vi "CalculateDependencies.vi"(6 "additional included files":path[](array[path]), 8 "error in (no error)":errorcluster, 11 "Build in":refnum<class "AB_EXE.lvclass">) -> (0 "error out":errorcluster, 2 "Dependencies":T1[](array[typedef]), 3 "Build out":refnum<class "AB_EXE.lvclass">)   [LabVIEW 2020, in "AB_EXE.lvclass"]
uses:
  <vilib>/AppBuilder/AB_Classes/EXE/AB_EXE.lvclass
  e:/builds/penguin/labview/branches/2020/dev/dist/vi.lib/AppBuilder/AB_Classes/Build/AB_Build.lvclass
  <vilib>/AppBuilder/AB_Dependency.ctl
  <vilib>/Utility/lvfile.llb/LVFileType.ctl
  <vilib>/AppBuilder/AB_Classes/EXE/AB_EXE.lvclass/AB_EXE.ctl
  <vilib>/AppBuilder/AB_Classes/EXE/AB_EXE_SharedVar_LibInfo.ctl
  <vilib>/AppBuilder/AB_Classes/Application/AB_Application.lvclass
  <vilib>/AppBuilder/AB_Classes/Build/AB_Build.lvclass
  <vilib>/Utility/lvfile.llb/NI_FileType.lvlib
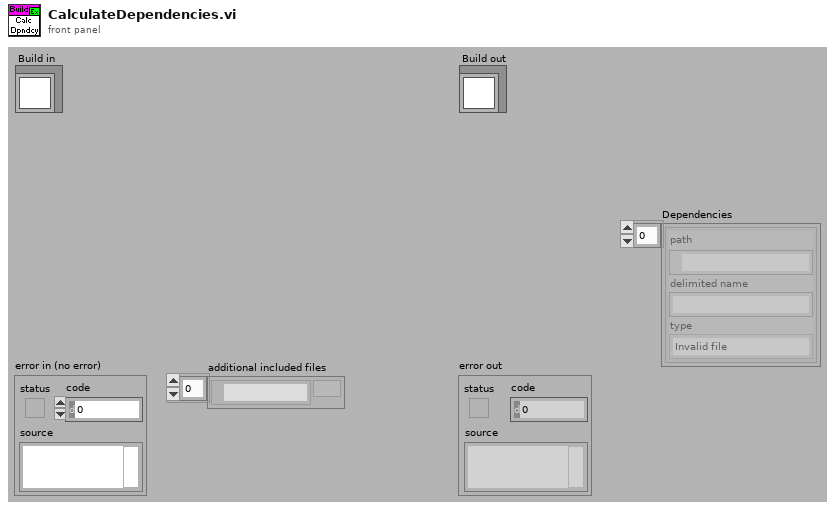
[diagram p1: front panel]
types:
  T1 = typedef "AB_Dependency.ctl" = cluster{"path":path, "delimited name":string, "type":T2}
  T2 = typedef "NI_FileType.lvlib/LVFileType.ctl" = enum32{"Invalid file", "Unknown type", "Instrument", "Control", "Polymorphic VI", "Project", "Library", "LVClass", "XControl", "XNode", "Shared library", ".NET assembly", "ActiveX interface", "CIN", "Run-time menu", "Palette menu", "Help file", "LLB", "XNode Edit Dependency", "Class Private Data Control", "Statechart", "MathScript .m file", "Ladder Diagram", "LVLibp", "XNode Build Dependency"}
  T3 = typedef "AB_EXE_SharedVar_LibInfo.ctl" = cluster{"LibraryPath":path, "LibraryItemID":string, "target":string, "deploy":bool}
  T4 = typedef "AB_Build.ctl" = cluster{"buildSpecName":string, "buildSpecDescription":string, "destinations":refnum<class "AB_Destination.lvclass">[], "exclusionOption":T5, "defaultLanguage":string, "supportedLanguages":string[], "excludedDirectories":path[], "buildContext":refnum<vi>, "buildObject":T6, "preview":bool, "programatic":bool, "progressBarEvents":T7, "userLog_Path":path, "preActionID":string, "preAction_Path":path, "postActionID":string, "postAction_Path":path, "eng_checkForBrokenVIs?":bool, "eng_verboseLinkerErrors?":bool, "localDest_Path":path, "targetDest_Path":path, "removeVIObject":u16, "cache":refnum<class "PreviewCache.lvclass">, "use cache":bool, "previewCache_ID":string, "buildCache_ID":string, "eng_TempLocalDest_Path":path, "eng_collectDependencies?":bool, "versionInfo":cluster{"buildVersion":cluster{"major":u16, "minor":u16, "patch":u16, "build":u16}, "autoIncrement":bool}, "eng_enableVIChecksums":bool}
  T5 = typedef "AB_Exclusion_Option.ctl" = cluster{"typedefs":bool, "polymorphicVIs":bool, "unusedLibraryItems":bool, "modifyLibraryFile":bool, "edit-timeDependencies":bool, "inlineVIs":bool, "dependent PPLs":bool, "dependent DLLs":bool}
  T6 = typedef "ItemRef.ctl" = u64
  T7 = typedef "provcom_ProgressBar_Events.ctl" = cluster{"newJob":refnum<user-event>, "newItem":refnum<user-event>, "errorMsg":T8, "cancel":refnum<user-event>}
  T8 = typedef "mxLvBuildError.ctl" = refnum<user-event>
  T9 = typedef "AB_Engine_RTDEP_Dep_Lib_Info.ctl" = cluster{"Library Path":path, "Target Name":string}
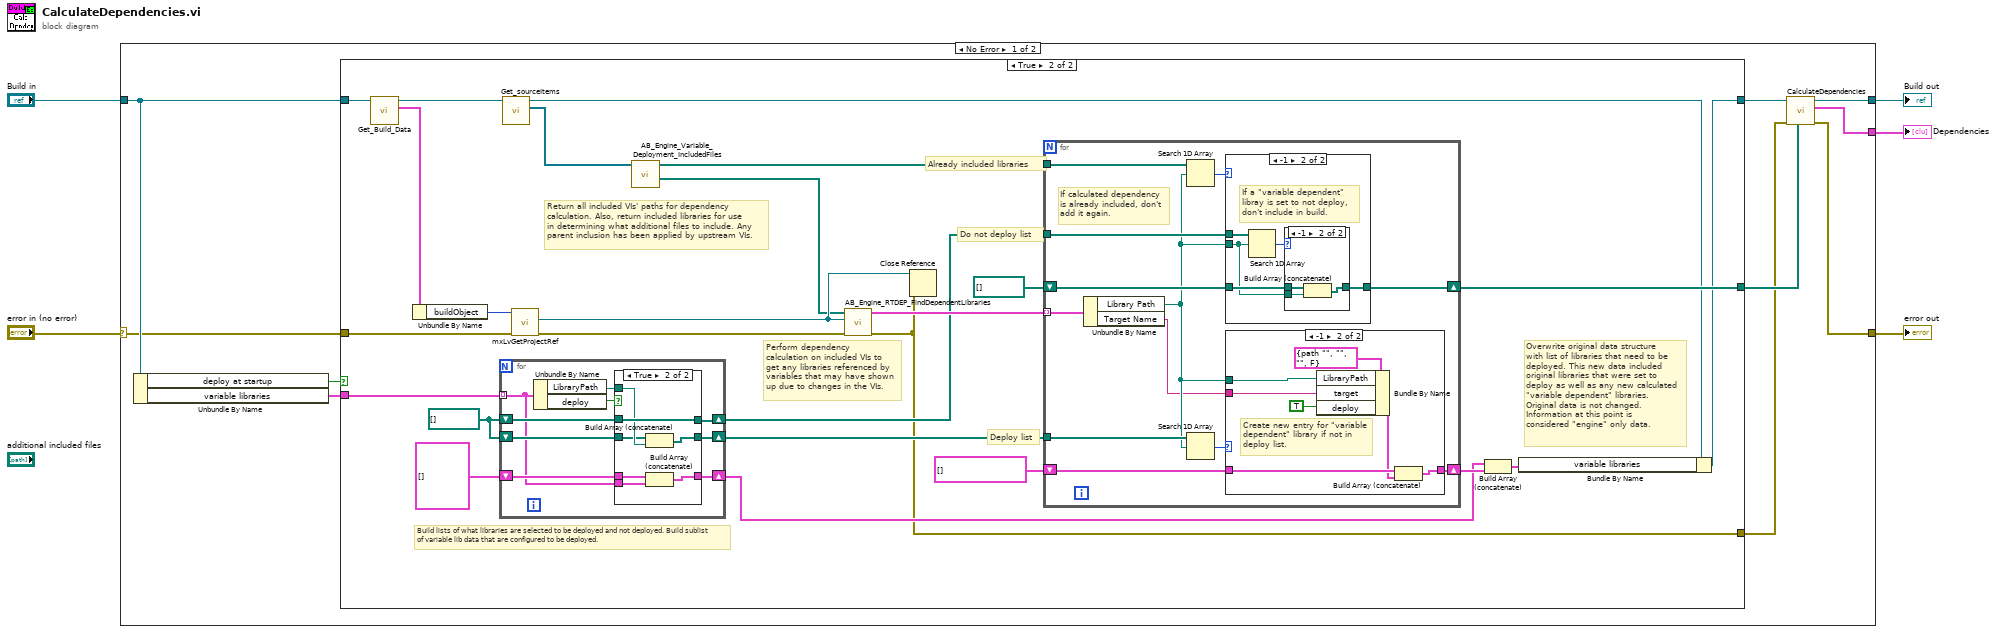
[diagram p0: block diagram]
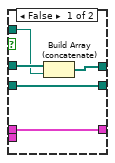
[diagram p3: hidden frame]
diagram:
  n1 = case shown="No Error" "error in (no error)" {
    selector: "error in (no error)" -> [w7 w95]
    tunnel: [w15 w95] -> w5
    tunnel: [w14 w94] -> w4
    tunnel: "Build in" -> [w12 w94]
    tunnel: [w6 _] -> w1
    frame No Error {
      n2 = Unbundle By Name(w12) -> ("deploy at startup"=w13:bool, "variable libraries"=w10:T3[])
      n3 = case shown="True" w13 {
        tunnel: w12 -> [w17 w42]
        tunnel: [w17 w28] -> w11
        tunnel: w10 -> [_ w26]
        tunnel: [_ w36] -> w9
        tunnel: w7 -> [w16 w23]
        tunnel: [w16 w18] -> w8
        frame False {
        }
        frame True {
          w34 = path[] []
          # "Overwrite original data structure with list of libraries that need to be deployed. This new data included original libraries that were set to deploy as well as any new calculated \"variable dependent\" libraries. Original data is not changed. Information at this point is considered \"engine\" only data."
          # "Already included libraries"
          # "Return all included VIs' paths for dependency calculation. Also, return included libraries for use in determining what additional files to include. Any parent inclusion has been applied by upstream VIs."
          # "Perform dependency calculation on included VIs to get any libraries referenced by variables that may have shown up due to changes in the VIs."
          # "Build lists of what libraries are selected to be deployed and not deployed. Build sublist of variable lib data that are configured to be deployed."
          # "Do not deploy list"
          # "Deploy list"
          n4 = call <vilib>:"Get_Build_Data.vi"("Class in"=w42) -> ("data"=w40:T4, "Class out"=w41:refnum<class "AB_EXE.lvclass">)  [unwired: 1 in, 8 out]
          n5 = Unbundle By Name(w40) -> ("buildObject"=w39:T6)
          n6 = for {
            tunnel: w26 -> [w43] mode=indexing
            shift-right: [w50] -> w37
            shift-left: w34 -> [w49]
            shift-right: [w48] -> w33
            shift-left: w34 -> [w47]
            shift-right: [w44] -> w25
            shift-left: T3[] [] ("variable libraries") -> [w45]
            n7 = Unbundle By Name(w43) -> ("LibraryPath"=w46:path, "deploy"=w51:bool)
            n8 = case shown="True" w51 {
              tunnel: [w56 w63] -> w50
              tunnel: w49 -> [w55 w63]
              tunnel: w46 -> [w54 w62]
              tunnel: [w53 w61] -> w48
              tunnel: w47 -> [w53 w60]
              tunnel: w45 -> [w52 w59]
              tunnel: [w52 w58] -> w44
              tunnel: w43 -> [_ w57]
              frame False {
                n9 = Build Array (concatenate)(w55, w54) -> (w56:path[])
              }
              frame True {
                n10 = Build Array (concatenate)(w60, w62) -> (w61:path[])
                n11 = Build Array (concatenate)(w59, w57) -> (w58:T3[])
              }
            }
          }
          n12 = call <vilib>:"Get_sourceItems.vi"("Class in"=w41) -> ("sourceItems"=w21:refnum<class "AB_Source.lvclass">[], "Class out"=w29:refnum<class "AB_EXE.lvclass">)  [unwired: 1 in, 8 out]
          n13 = call <resource>:"mxLvGetProjectRef.vi"("error in"=w23, "Item"=w39) -> ("error out"=w22:errorcluster, "Project Refnum"=w35:refnum<vi>)  [unwired: 8 out]
          n14 = call <vilib>:"AB_Engine_Variable_Deployment_IncludedFiles.vi"("source items"=w21) -> ("Included VIs"=w19:path[], "Included libraries"=w20:path[])  [unwired: 2 in, 7 out]
          n15 = call <vilib>:"AB_Engine_RTDEP_FindDependentLibraries.vi"("error in (no error)"=w22, "Project Refnum"=w35, "included files"=w19) -> ("error out"=w18:errorcluster, "Dependent Library Path Array"=w38:T9[])  [unwired: 1 in, 6 out]
          n16 = Close Reference(reference=w35, error in (no error)=w18) -> ()  [unwired: 1 out]
          n17 = for {
            tunnel: w38 -> [w75] mode=indexing
            tunnel: w37 -> [w74]
            shift-right: [w73] -> w36
            shift-left: path[] [] -> [w72]
            tunnel: w20 -> [w71]
            tunnel: w33 -> [w69]
            shift-right: [w66] -> w31
            shift-left: T3[] [] ("variable libraries") -> [w67]
            # "If calculated dependency is already included, don't add it again."
            n18 = Unbundle By Name(w75) -> ("Library Path"=w65:path, "Target Name"=w64:string)
            n19 = Search 1D Array(1D array=w71, element=w65) -> (index of element=w70:i32)  [unwired: 1 out]
            n20 = Search 1D Array(1D array=w69, element=w65) -> (index of element=w68:i32)  [unwired: 1 out]
            n21 = case shown="-1" w70 {
              tunnel: w74 -> [_ w89]
              tunnel: [w84 w87] -> w73
              tunnel: w72 -> [w84 w86]
              tunnel: w65 -> [_ w85]
              frame Default {
              }
              frame -1 {
                # "If a \"variable dependent\" libray is set to not deploy, don't include in build."
                n22 = Search 1D Array(1D array=w89, element=w85) -> (index of element=w88:i32)  [unwired: 1 out]
                n23 = case shown="-1" w88 {
                  tunnel: w85 -> [_ w93]
                  tunnel: [w90 w92] -> w87
                  tunnel: w86 -> [w90 w91]
                  frame Default {
                  }
                  frame -1 {
                    n24 = Build Array (concatenate)(w91, w93) -> (w92:path[])
                  }
                }
              }
            }
            n25 = case shown="-1" w68 {
              tunnel: w67 -> [w76 w83]
              tunnel: [w76 w82] -> w66
              tunnel: w65 -> [_ w78]
              tunnel: w64 -> [_ w77]
              frame Default {
              }
              frame -1 {
                # "Create new entry for \"variable dependent\" library if not in deploy list."
                n26 = Bundle By Name(cluster=T3 {"LibraryPath"=path "", "LibraryItemID"="", "target"="", "deploy"=FALSE} ("variable lib"), "LibraryPath"=w78, "target"=w77, "deploy"=TRUE) -> (w79:T3)
                n27 = Build Array (concatenate)(w83, w79) -> (w82:T3[])
              }
            }
          }
          n28 = Build Array (concatenate)(w25, w31) -> (w30:T3[])
          n29 = Bundle By Name(cluster=w29, "variable libraries"=w30) -> (w28:refnum<class "AB_EXE.lvclass">)
        }
      }
      n30 = call-parent "CalculateDependencies.vi"("additional included files"=w9, "error in (no error)"=w8, "Build in"=w11) -> ("error out"=w15:errorcluster, "Dependencies"=w6:T1[], "Build out"=w14:refnum<class "AB_EXE.lvclass">)  [unwired: 6 out]
    }
    frame Error {
    }
  }
  "error out" <- w5
  "Build out" <- w4
  "Dependencies" <- w1
